vi "RT Driver VI.vi"(6 "Device Clock":string, 9 "Device Inputs FIFO":refnum<k33>, 10 "Device Outputs FIFO":refnum<k33>, 11 "Device Reference":T1 format="%.0x") -> ()   [LabVIEW 2016, in "UDP Sender Engine.lvlib"]
uses:
  UDP Sender Engine.lvlib
  <vilib>/NI Veristand/Custom Device API/Custom Device Item Ref.ctl
  <vilib>/NI Veristand/Custom Device API/Custom Device Channel Type.ctl
  Shared/Constants.vi
  <vilib>/NI Veristand/Custom Device API/Custom Device API.lvlib
  <vilib>/NI Veristand/Custom Device Tools/Custom Device Utility Library/Custom Device Utility Library.lvlib
  Shared/UDP Sender Shared.lvlib
panel:
  in  "Initialization Status Notifier":refnum<notifier>
  in  "Status Notifier":refnum<notifier>
  # "Custom Device Template\nv1.0"
  # "Use this template as a starting point for creating a custom device code module. The input controls shown here are specially named controls that the system will use to provide the device loop with data. The controls are not required for the device loop to run. For instance, if the device doesn't produce any output data, then you don't need the Device Outputs FIFO control. If you do use these controls, however, they need to have these exact names to be functional."
  # "The optional status notifier element is used to notify the RT engine of the last state of the custom device, and to indicate the device has completed execution. If this control is not used, a default No Error value is returned to the system when the device finishes execution.\n\nNote: This error state is not checked until the system shuts down. Use an output status channel to send more immediate status values to the system."
  # "This optional input can be used to send the VeriStand Engine the final status of the custom device initalization process. If this control exists on the custom device front panel, the VeriStand Engine will wait for a status update before starting up. If the custom device reports an error, that will abort the execution of the current configuration in the VeriStand Engine.\n\nThis control can be deleted if the custom device does not need to send the initialization status update."
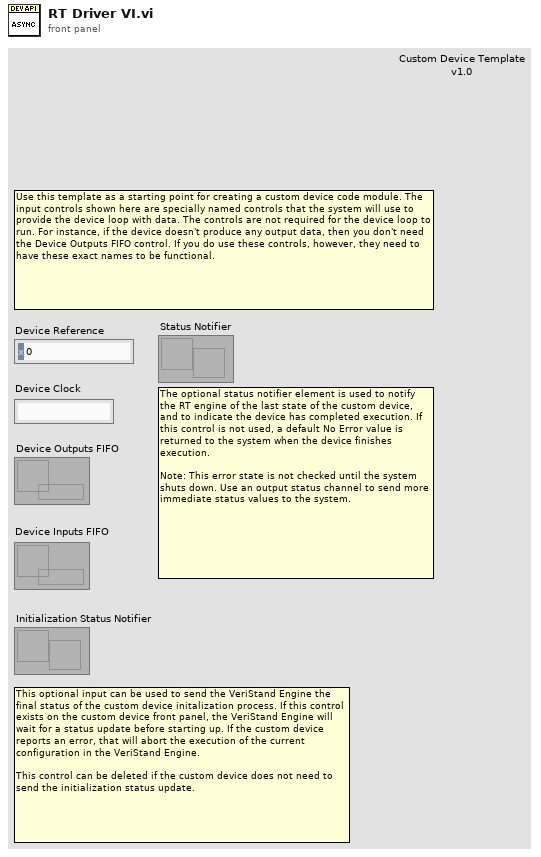
[diagram p1: front panel]
types:
  T1 = typedef "Custom Device API.lvlib/Custom Device Item Ref.ctl" = u64
  T2 = typedef "Custom Device API.lvlib/Custom Device Channel Type.ctl" = enum16{"Input", "Output"}
  T3 = typedef "Custom Device API.lvlib/Custom Device Engine Event Ref.ctl" = refnum<event-registration>
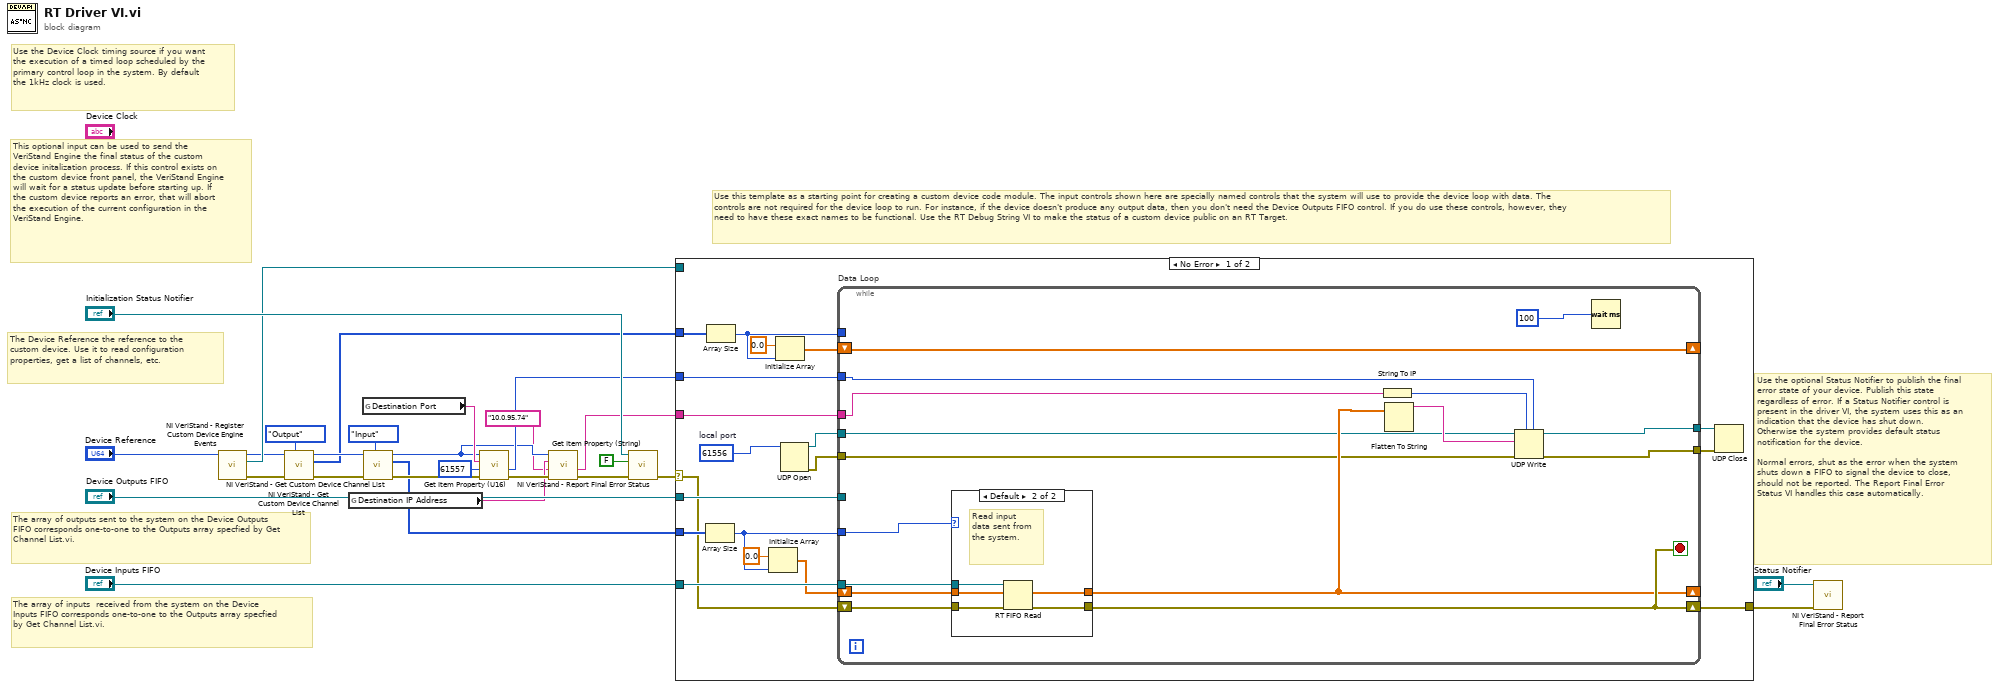
[diagram p0: block diagram]
diagram:
  # "This optional input can be used to send the VeriStand Engine the final status of the custom device initalization process. If this control exists on the custom device front panel, the VeriStand Engine will wait for a status update before starting up. If the custom device reports an error, that will abort the execution of the current configuration in the VeriStand Engine."
  # "The array of inputs  received from the system on the Device Inputs FIFO corresponds one-to-one to the Outputs array specfied by Get Channel List.vi."
  # "Use the optional Status Notifier to publish the final error state of your device. Publish this state regardless of error. If a Status Notifier control is present in the driver VI, the system uses this as an indication that the device has shut down. Otherwise the system provides default status notification for the device.\n\nNormal errors, shut as the error when the system shuts down a FIFO to signal the device to close, should not be reported. The Report Final Error Status VI handles this case automatically."
  # "The array of outputs sent to the system on the Device Outputs FIFO corresponds one-to-one to the Outputs array specfied by Get Channel List.vi."
  # "The Device Reference the reference to the custom device. Use it to read configuration properties, get a list of channels, etc."
  # "Use the Device Clock timing source if you want the execution of a timed loop scheduled by the primary control loop in the system. By default the 1kHz clock is used."
  # "Use this template as a starting point for creating a custom device code module. The input controls shown here are specially named controls that the system will use to provide the device loop with data. The controls are not required for the device loop to run. For instance, if the device doesn't produce any output data, then you don't need the Device Outputs FIFO control. If you do use these controls, however, they need to have these exact names to be functional. Use the RT Debug String VI to make the status of a custom device public on an RT Target."
  n1 = call <vilib>:"NI VeriStand - Register Custom Device Engine Events.vi"("Device Ref in"="Device Reference") -> ("error out"=w27:errorcluster, "Custom Device Engine Event Ref"=w15:T3, "Device Ref out"=w12:T1)  [unwired: 8 in]
  n2 = call <vilib>:"NI VeriStand - Get Custom Device Channel List.vi"("Channel Type"=Custom_Device_Channel_Type."Output", "error in (no error)"=w27, "Device Ref in"=w12) -> ("error out"=w20:errorcluster, "Specified Channel Ref List"=w17:T1[], "Device Ref out"=w21:T1)  [unwired: 6 out]
  n3 = global read "Constants.vi" "Destination IP Address"() -> (w6:string)
  n4 = global read "Constants.vi" "Destination Port"() -> (w7:string)
  n5 = call <vilib>:"NI VeriStand - Get Custom Device Channel List.vi"("Channel Type"=Custom_Device_Channel_Type."Input", "error in (no error)"=w20, "Device Ref in"=w21) -> ("error out"=w26:errorcluster, "Specified Channel Ref List"=w18:T1[], "Device Ref out"=w3:T1)  [unwired: 6 out]
  n6 = call <vilib>:"Get Item Property (U16).vi"("error in (no error)"=w26, "Default Value"=u16 61557, "Property Name"=w7, "Item Ref in"=w3) -> ("error out"=w8:errorcluster, "Value"=w5:u16)  [unwired: 4 in, 2 out]
  n7 = call <vilib>:"Get Item Property (String).vi"("error in (no error)"=w8, "Default Value"="10.0.95.74", "Property Name"=w6, "Item Ref in"=w3) -> ("error out"=w9:errorcluster, "Value"=w4:string)  [unwired: 4 in, 2 out]
  n8 = call <vilib>:"NI VeriStand - Report Final Error Status.vi"("error in (no error)"=w9, "Filter FIFO & Shutdown Errors (T)"=FALSE ("Filter FIFO Errors (T)"), "Status Notifier"="Initialization Status Notifier") -> ("error out"=w11:errorcluster)  [unwired: 8 out]
  n9 = case shown="No Error" w11 {
    selector: w11 -> [w36 w70]
    tunnel: "Device Outputs FIFO" -> [w46 _]
    tunnel: "Device Inputs FIFO" -> [w45 _]
    tunnel: w18 -> [w39 _]
    tunnel: w17 -> [w38 _]
    tunnel: w15 -> [_ _]
    tunnel: [w35 w70] -> w14
    tunnel: w5 -> [w34 _]
    tunnel: w4 -> [w33 _]
    frame No Error {
      w32 = u16 61556  # local port
      n10 = Array Size(array=w39) -> (size(s)=w37:i32)
      n11 = Array Size(array=w38) -> (size(s)=w40:i32)
      n12 = Initialize Array(0.0 ("element"), w37) -> (w41:dbl[])
      n13 = Initialize Array(0.0 ("element"), w40) -> (w42:dbl[])
      n14 = UDP Open(11:w32) -> (port=w31:refnum<k16>, 0:w30:errorcluster)  [unwired: 4 in, 1 out]
      n15 = while "Data Loop" {
        shift-right: [w53] -> _
        shift-left: w41 -> [w61]
        shift-right: [w56] -> w35
        shift-left: w36 -> [w62]
        shift-right: [w60] -> _
        shift-left: w42 -> [w60]
        tunnel: w40 -> [_]
        tunnel: w46 -> [_]
        tunnel: w45 -> [w59]
        tunnel: w37 -> [w58]
        tunnel: w34 -> [w51]
        tunnel: w33 -> [w52]
        tunnel: w31 -> [w50]
        tunnel: w30 -> [w49]
        tunnel: [w48] -> w29
        tunnel: [w47] -> w28
        stop <- w56 stop-if-true
        n16 = case shown="Default" w58 {
          tunnel: w59 -> [_ w69]
          tunnel: w61 -> [w64 w68]
          tunnel: [w64 w67] -> w53
          tunnel: [w63 w66] -> w56
          tunnel: w62 -> [w63 w65]
          frame 0 {
            # "No inputs to read\nfrom system. Inputs FIFO not created in this case, so don't write to it."
          }
          frame Default {
            # "Read input data sent from the system."
            n17 = RT FIFO Read(0:w69, 1:w68, 3:w65) -> (9:w67:dbl[], 11:w66:errorcluster)  [unwired: 4 out]
          }
        }
        n18 = String To IP(1:w52) -> (0:w55:u32)
        n19 = Flatten To String(anything=w53) -> (data string=w54:string)  [unwired: 3 in, 2 out]
        n20 = UDP Write(address=w55, port or service name=w51, connection ID=w50, data in=w54, 8:w49) -> (error out=w47:errorcluster, 3:w48:refnum<k16>)  [unwired: 1 in]
        n21 = Wait (ms)(milliseconds to wait=u32 100) -> ()  [unwired: 1 out]
      }
      n22 = UDP Close(connection ID=w29, 8:w28) -> ()  [unwired: 2 out]
    }
    frame Error {
    }
  }
  n23 = call <vilib>:"NI VeriStand - Report Final Error Status.vi"("error in (no error)"=w14, "Status Notifier"="Status Notifier") -> ()  [unwired: 1 in, 9 out]
